vi "TimeAndTemperature (SubVI).vi"(8 "error in (no error)":errorcluster, 10 "Command":string="FETC?", 11 "GPIB Address: Temperature":string="16") -> (0 "error out":errorcluster, 1 "Temp":dbl, 2 "double( Time, Temp )":dbl[](array[numeric]), 3 "str( Time, Temp )":string[](array[string]))   [LabVIEW 2016]
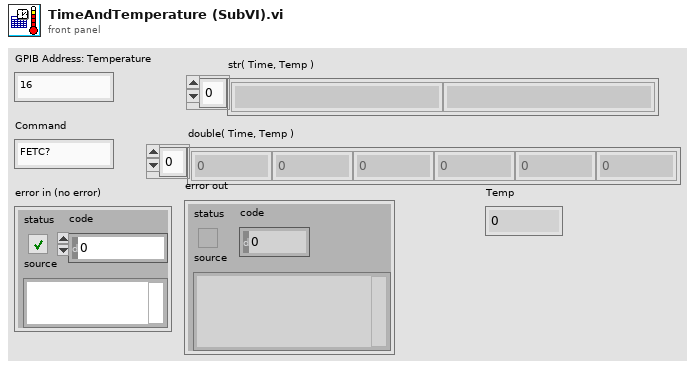
[diagram p1: front panel]
types:
  T1 = typedef "LVDateTimeRec.ctl" = cluster{"fractional second":dbl, "second":i32, "minute":i32, "hour":i32, "day of month":i32, "month":i32, "year":i32, "day of week":i32, "day of year":i32, "DST":i32}
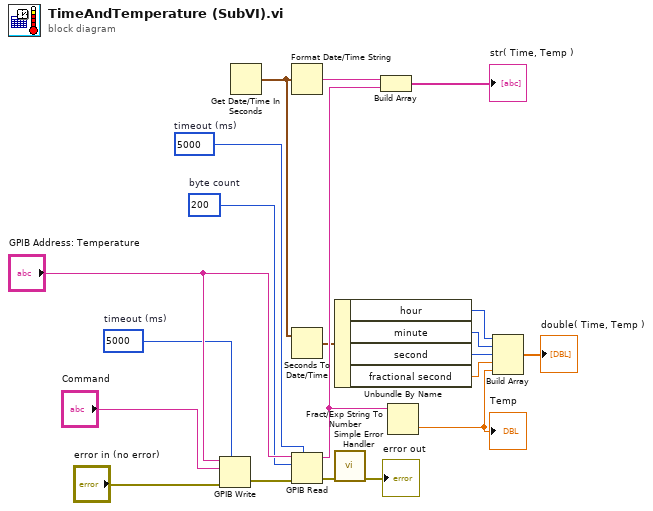
[diagram p0: block diagram]
diagram:
  w8 = 5000  # timeout (ms)
  w5 = 200  # byte count
  w6 = 5000  # timeout (ms)
  n1 = GPIB Write(0:"GPIB Address: Temperature", 1:"Command", 3:"error in (no error)", 4:w6) -> (6:w2:errorcluster)  [unwired: 1 in, 1 out]
  n2 = Get Date/Time In Seconds() -> (seconds since 1Jan1904=w9:timestamp)
  n3 = Format Date/Time String(seconds (now)=w9) -> (date/time string=w11:string)  [unwired: 2 in]
  n4 = Seconds To Date/Time(time stamp (now)=w9) -> (date time rec=w10:T1)  [unwired: 1 in]
  n5 = GPIB Read(0:"GPIB Address: Temperature", 1:w5, 3:w2, 4:w8) -> (5:w12:string, 7:w3:errorcluster)  [unwired: 1 in, 1 out]
  n6 = Unbundle By Name(w10) -> ("hour"=w14:i32, "minute"=w15:i32, "second"=w16:i32, "fractional second"=w17:dbl)
  n7 = call <vilib>:"Simple Error Handler.vi"("error in (no error)"=w3) -> ("error out"=→"error out":errorcluster)  [unwired: 4 in, 4 out]
  n8 = Build Array(w11, w12) -> (→"str( Time, Temp )":string[])
  n9 = Fract/Exp String To Number(string=w12) -> (number=w19:dbl)  [unwired: 3 in, 1 out]
  "Temp" <- w19
  n10 = Build Array(w14, w15, w16, w17, w19) -> (→"double( Time, Temp )":dbl[])
